vi "Introspection Core.vi"(8 "error in (no error)":errorcluster, 11 "CS++DCPwr in":refnum<class "CS++DCPwr.lvclass">) -> (0 "error out":errorcluster, 2 "CS++Messages":refnum<class "Message.lvclass">[](array[class]), 3 "CS++DCPwr out":refnum<class "CS++DCPwr.lvclass">)   [LabVIEW 2015, in "CS++DCPwr.lvlib" / "CS++DCPwr.lvclass"]
doc: "This vi delivers a list with all messages this actor reacts to. \n\nNote that all inherited classes have to overwrite it."
uses:
  CS++DCPwr.lvclass
  <vilib>/ActorFramework/Message/Message.lvclass
  CS++DCPwr Messages/Get Channel Name Msg/Get Channel Name Msg.lvclass
  CS++DCPwr Messages/Query Max Current Limit Msg/Query Max Current Limit Msg.lvclass
  CS++DCPwr Messages/Query Max Voltage Level Msg/Query Max Voltage Level Msg.lvclass
  CS++DCPwr Messages/Query Output State Msg/Query Output State Msg.lvclass
  CS++DCPwr Messages/Configure Trigger Source [TRG] Msg/Configure Trigger Source [TRG] Msg.lvclass
  CS++DCPwr Messages/Configure Triggered Voltage Level [TRG] Msg/Configure Triggered Voltage Level [TRG] Msg.lvclass
  CS++DCPwr Messages/Configure Triggered Current Limit [TRG] Msg/Configure Triggered Current Limit [TRG] Msg.lvclass
  CS++DCPwr Messages/Configure Output Enable Msg/Configure Output Enable Msg.lvclass
  CS++DCPwr Messages/Configure Output Range Msg/Configure Output Range Msg.lvclass
  CS++DCPwr Messages/Configure Current Limit Msg/Configure Current Limit Msg.lvclass
  CS++DCPwr Messages/Configure OVP Msg/Configure OVP Msg.lvclass
  CS++DCPwr Messages/Configure Voltage Level Msg/Configure Voltage Level Msg.lvclass
  CS++DCPwr Messages/Configure Desired Output State Msg/Configure Desired Output State Msg.lvclass
  CS++DCPwr Messages/Initiate [TRG] Msg/Initiate [TRG] Msg.lvclass
  CS++DCPwr Messages/Send Software Trigger [SWT] Msg/Send Software Trigger [SWT] Msg.lvclass
  CS++DCPwr Messages/Abort [TRG] Msg/Abort [TRG] Msg.lvclass
  CS++DCPwr Messages/Reset Output Protection Msg/Reset Output Protection Msg.lvclass
  CS++DCPwr Messages/Measure [MSR] Msg/Measure [MSR] Msg.lvclass
  CSPP_Core/Actors/CS++DeviceActor/CS++DeviceActor.lvclass
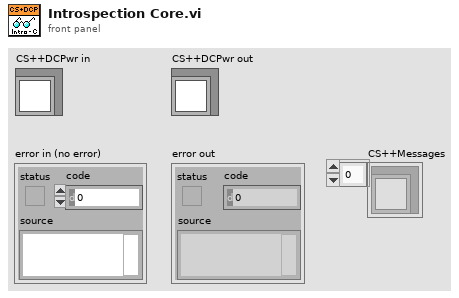
[diagram p1: front panel]
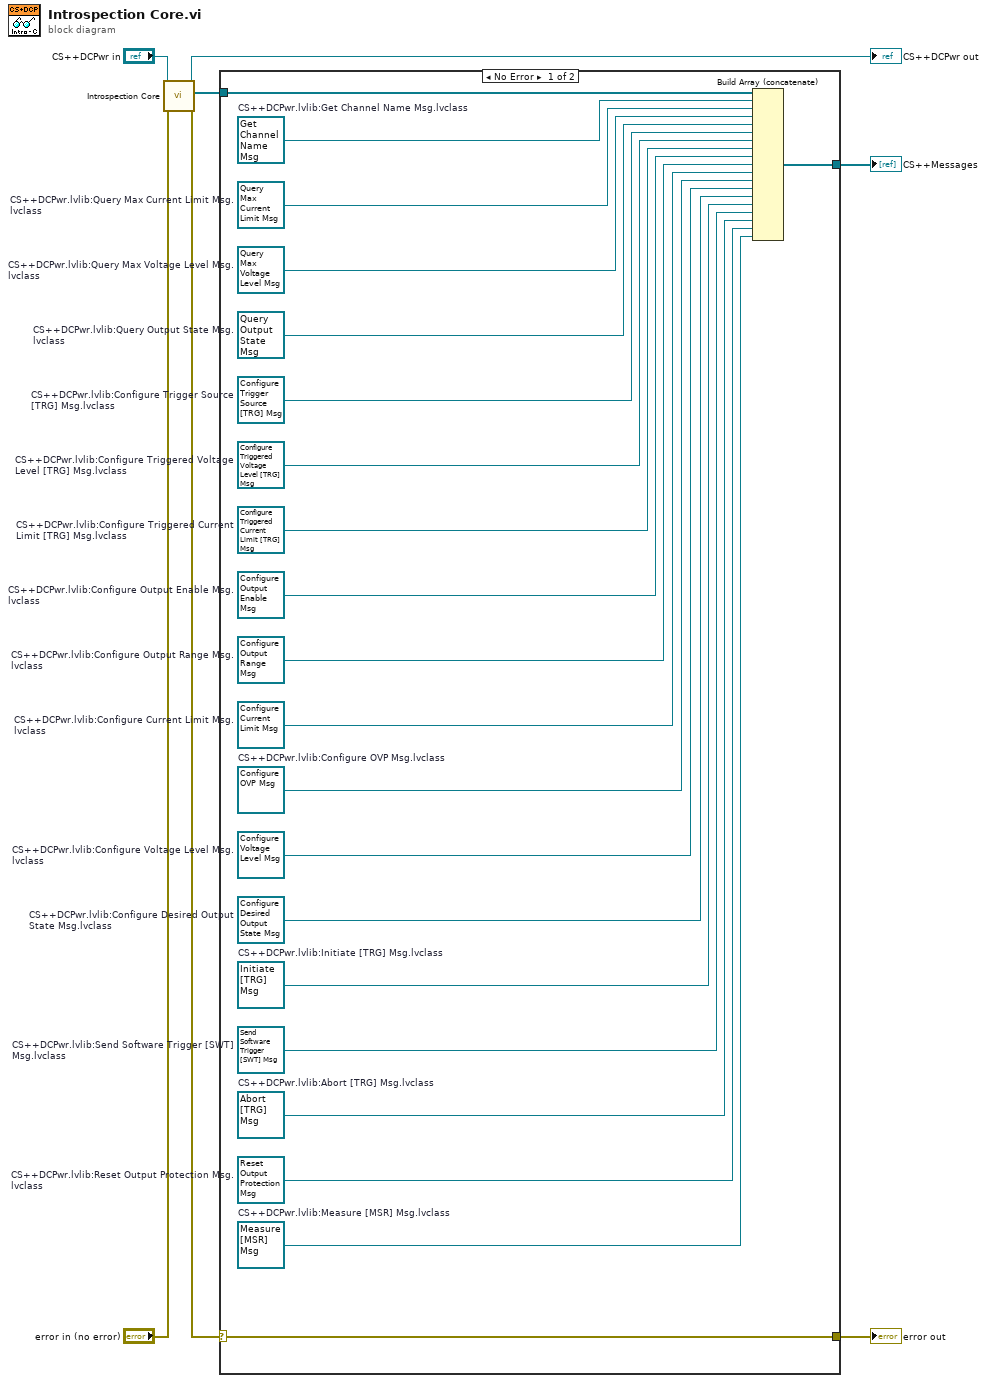
[diagram p0: block diagram]
diagram:
  n1 = call-parent "Introspection Core.vi"("error in (no error)"="error in (no error)", "CS++DeviceActor in"="CS++DCPwr in") -> ("error out"=w4:errorcluster, "CS++Messages"=w2:refnum<class "Message.lvclass">[], "CS++DeviceActor out"=→"CS++DCPwr out":refnum<class "CS++DCPwr.lvclass">)  [unwired: 7 in]
  n2 = case shown="No Error" w4 {
    selector: w4 -> [w28 w29]
    tunnel: [w28 w29] -> w3
    tunnel: w2 -> [w27 _]
    tunnel: [w8 _] -> w1
    frame No Error {
      w9 = refnum<class "Measure [MSR] Msg.lvclass"> refnum  # CS++DCPwr.lvlib:Measure [MSR] Msg.lvclass
      w10 = refnum<class "Reset Output Protection Msg.lvclass"> refnum  # CS++DCPwr.lvlib:Reset Output Protection Msg.lvclass
      w11 = refnum<class "Abort [TRG] Msg.lvclass"> refnum  # CS++DCPwr.lvlib:Abort [TRG] Msg.lvclass
      w12 = refnum<class "Send Software Trigger [SWT] Msg.lvclass"> refnum  # CS++DCPwr.lvlib:Send Software Trigger [SWT] Msg.lvclass
      w13 = refnum<class "Initiate [TRG] Msg.lvclass"> refnum  # CS++DCPwr.lvlib:Initiate [TRG] Msg.lvclass
      w14 = refnum<class "Configure Desired Output State Msg.lvclass"> refnum  # CS++DCPwr.lvlib:Configure Desired Output State Msg.lvclass
      w15 = refnum<class "Configure Voltage Level Msg.lvclass"> refnum  # CS++DCPwr.lvlib:Configure Voltage Level Msg.lvclass
      w16 = refnum<class "Configure OVP Msg.lvclass"> refnum  # CS++DCPwr.lvlib:Configure OVP Msg.lvclass
      w17 = refnum<class "Configure Current Limit Msg.lvclass"> refnum  # CS++DCPwr.lvlib:Configure Current Limit Msg.lvclass
      w18 = refnum<class "Configure Output Range Msg.lvclass"> refnum  # CS++DCPwr.lvlib:Configure Output Range Msg.lvclass
      w19 = refnum<class "Configure Output Enable Msg.lvclass"> refnum  # CS++DCPwr.lvlib:Configure Output Enable Msg.lvclass
      w20 = refnum<class "Configure Triggered Current Limit [TRG] Msg.lvclass"> refnum  # CS++DCPwr.lvlib:Configure Triggered Current Limit [TRG] Msg.lvclass
      w21 = refnum<class "Configure Triggered Voltage Level [TRG] Msg.lvclass"> refnum  # CS++DCPwr.lvlib:Configure Triggered Voltage Level [TRG] Msg.lvclass
      w22 = refnum<class "Configure Trigger Source [TRG] Msg.lvclass"> refnum  # CS++DCPwr.lvlib:Configure Trigger Source [TRG] Msg.lvclass
      w23 = refnum<class "Query Output State Msg.lvclass"> refnum  # CS++DCPwr.lvlib:Query Output State Msg.lvclass
      w24 = refnum<class "Query Max Voltage Level Msg.lvclass"> refnum  # CS++DCPwr.lvlib:Query Max Voltage Level Msg.lvclass
      w25 = refnum<class "Query Max Current Limit Msg.lvclass"> refnum  # CS++DCPwr.lvlib:Query Max Current Limit Msg.lvclass
      w26 = refnum<class "Get Channel Name Msg.lvclass"> refnum  # CS++DCPwr.lvlib:Get Channel Name Msg.lvclass
      n3 = Build Array (concatenate)(w27, w26, w25, w24, w23, w22, w21, w20, w19, w18, w17, w16, w15, w14, w13, w12, w11, w10, w9) -> (w8:refnum<class "Message.lvclass">[])
    }
    frame Error {
    }
  }
  "error out" <- w3
  "CS++Messages" <- w1
